vi "ProjectedLanding.vi"(10 "ProjectedPosition":cluster{dbl, dbl}, 11 "Image In":T1) -> (3 "Image Out":T1)   [LabVIEW 2012]
uses:
  <vilib>/vision/Image Controls.llb/IMAQ Image.ctl
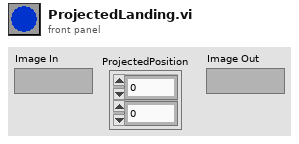
[diagram p1: front panel]
types:
  T1 = typedef "IMAQ Image.ctl" = refnum<image>
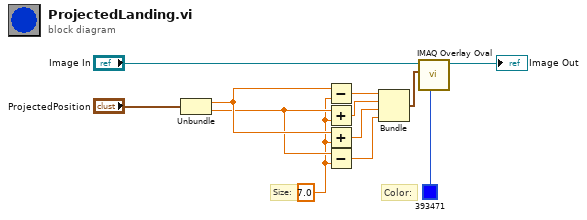
[diagram p0: block diagram]
diagram:
  w1 = 7.0 ("y")
  # "Color:"
  # "Size:"
  n1 = Unbundle("ProjectedPosition") -> (w6:dbl, w5:dbl)
  n2 = Subtract(x=w6, y=w1) -> (x-y=w11:dbl)
  n3 = Add(x=w5, y=w1) -> (x+y=w12:dbl)
  n4 = Add(x=w6, y=w1) -> (x+y=w10:dbl)
  n5 = Subtract(x=w5, y=w1) -> (x-y=w9:dbl)
  n6 = Bundle(w11, w12, w10, w9) -> (w7:cluster{dbl, dbl, dbl, dbl})  [unwired: 1 in]
  n7 = call "IMAQ Overlay Oval"("Color"=u32 393471, "Bounding Rectangle"=w7, "Image"="Image In") -> ("Image Out"=→"Image Out":T1)  [unwired: 7 in, 1 out]
